vi "Test - Check for Definition.vi"   [LabVIEW 2023, in "JSON Schema Generator.lvlib"]
uses:
  JSON Schema Generator.lvlib
  Defintion FGV Actions.ctl
  <vilib>/addons/_JKI Toolkits/Caraya/classes/Assert/Assert Equal Value_Variant.vi
  <vilib>/addons/_JKI Toolkits/Caraya/classes/Assert/Assert Not Error.vi
  <vilib>/addons/_JKI Toolkits/Caraya/classes/Test/Test.lvclass
  <vilib>/addons/_JKI Toolkits/Caraya/classes/Assert/Assert.lvclass
types:
  T1 = typedef "JSON Schema Generator.lvlib/Defintion FGV Actions.ctl" = enum16{"Create Defs", "Update Defs", "Get all Defs", "Get Def"}
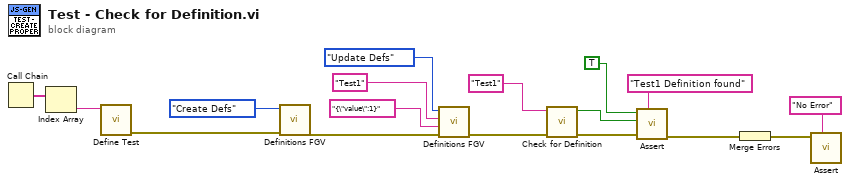
[diagram p0: block diagram]
diagram:
  n1 = Call Chain() -> (call chain=w17:string[])
  n2 = Index Array(array=w17) -> (element=w16:string)  [unwired: 1 in]
  n3 = call <vilib>:"Define Test.vi"("Label (VI Title)"=w16) -> ("error out"=w10:errorcluster)  [unwired: 9 in, 1 out]
  n4 = call "Definitions FGV.vi"("error in (no error)"=w10, "Action"=Defintion_FGV_Actions."Create Defs") -> ("error out"=w8:errorcluster)  [unwired: 7 in, 2 out]
  n5 = call "Definitions FGV.vi"("error in (no error)"=w8, "Defintion Schema In"="{\"value\":1}" ("Definition Schema"), "Definition Name"="Test1" ("Name"), "Action"=Defintion_FGV_Actions."Update Defs") -> ("error out"=w7:errorcluster)  [unwired: 5 in, 2 out]
  n6 = call "Check for Definition.vi"("error in (no error)"=w7, "Definition Name"="Test1") -> ("error out"=w3:errorcluster, "Found?"=w2:bool)  [unwired: 8 in]
  n7 = call-poly <vilib>:"Assert.vi"("Label"="Test1 Definition found", "error in (no error)"=w3, "Y"=w2, "X"=TRUE) -> ("error out"=w14:errorcluster)  [unwired: 6 in, 1 out]
  n8 = Merge Errors(w14) -> (w12:errorcluster)
  n9 = call-poly <vilib>:"Assert.vi"("Label"="No Error", "Not Error?"=w12) -> ()  [unwired: 8 in, 2 out]
